vi "Test MultiValue INSERT.vi"(9 "file (use dialog)":path, 10 "Method":T1(ring), 11 "Numeric":i32=1000000) -> (2 "Rows/sec":dbl format="%#_3p", 3 "Time per row":dbl format="%#_3p")   [LabVIEW 2016, in "LV-Data.PGSQL.lvclass"]
uses:
  LV-Data.PGSQL.lvclass
  <vilib>/JDP Science/PostgreSQL Library/Result/PQ Result.lvclass/PQ Result.ctl
  <vilib>/JDP Science/PostgreSQL Library/Connection/Execute Command (No results).vi
  <vilib>/JDP Science/PostgreSQL Library/Result/Clear.vi
  <vilib>/JDP Science/PostgreSQL Library/Connection/Execute Command (Result).vi
  <vilib>/JDP Science/PostgreSQL Library/Connection/Execute (no results).vi
  <vilib>/JDP Science/PostgreSQL Library/Connection/Execute (Return first result with rows).vi
  <vilib>/JDP Science/PostgreSQL Library/Connection/Single Command with parameters.vi
  <userlib>/_OpenG.lib/string/string.llb/Trim Whitespace (String)__ogtk.vi
  <vilib>/JDP Science/PostgreSQL Library/Connection/PQ Connection.lvclass
panel:
  out "concatenated string":string
  in  "Connection Strings to access PostgreSQL":string="host=localhost port=5432 dbname = mydb "
  out "error out":errorcluster
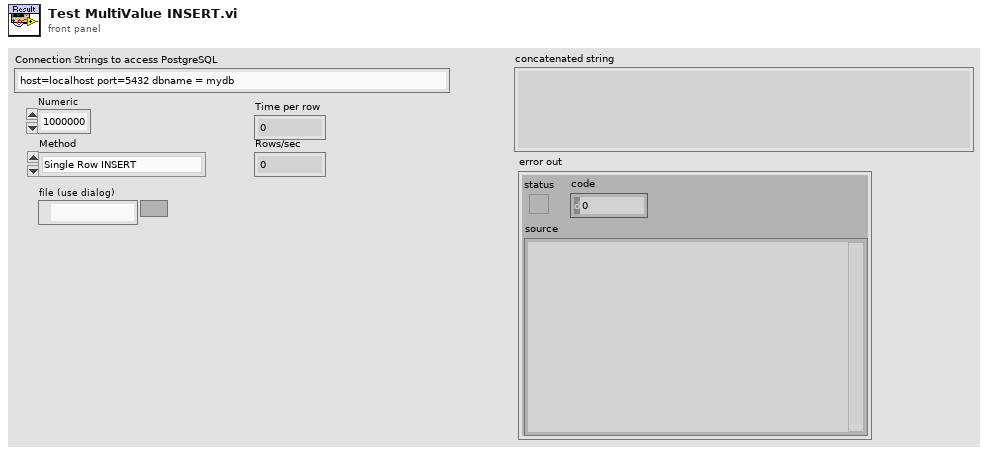
[diagram p1: front panel]
types:
  T1 = enum16{"Single Row INSERT", "Multi Row INSERT", "COPY", "COPY file"}
  T2 = cluster{i32, "number: 0 to 1":dbl, string, "seconds since 1Jan1904":timestamp}
  T3 = typedef "NI_Data Type.lvlib/Data Type.ctl" = enum8{"Invalid Type", "Void", "I8", "I16", "I32", "I64", "U8", "U16", "U32", "U64", "Single Float", "Double Float", "Extended Float", "Single Complex", "Double Complex", "Extended Complex", "Enum U8", "Enum U16", "Enum U32", "Enum U64", "Single Float With Unit", "Double Float With Unit", "Extended Float With Unit", "Single Complex with Unit", "Double Complex with Unit", "Extended Complex with Unit", "Boolean", "String", "Path", "Picture", "Tag", "Array", "Cluster", "Variant", "LV Variant", "Waveform", "Timestamp", "Digital Waveform", "Digital Data", "ExpressData", "Refnum", "External Data", "VI", "Poly VI", "LabVIEW Class Instance", "Fixed Point"}
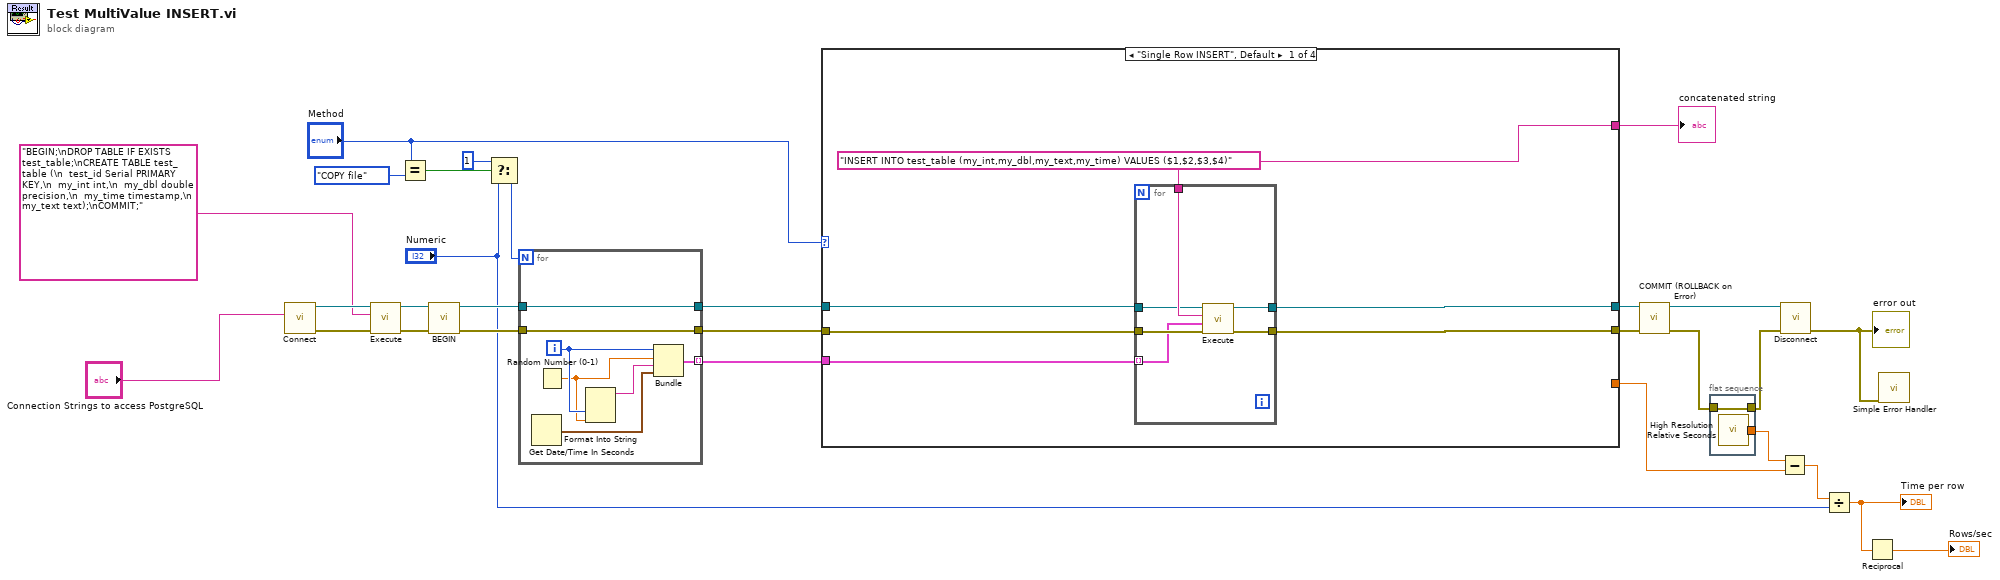
[diagram p0: block diagram]
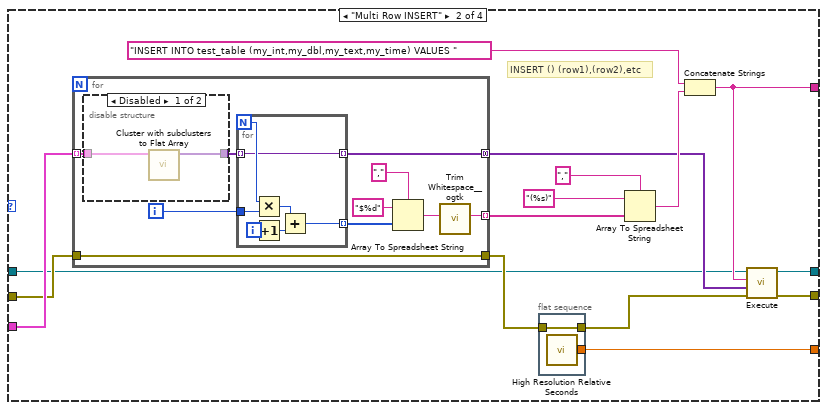
[diagram p2: hidden frame]
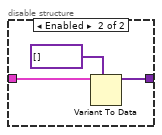
[diagram p3: hidden frame]
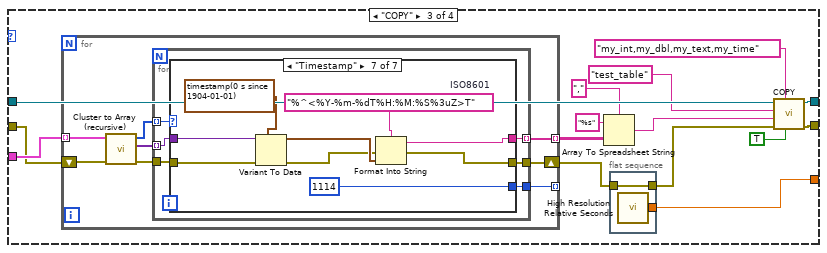
[diagram p4: hidden frame]
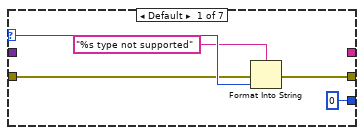
[diagram p5: hidden frame]
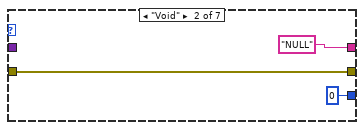
[diagram p6: hidden frame]
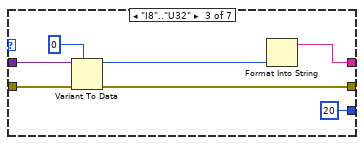
[diagram p7: hidden frame]
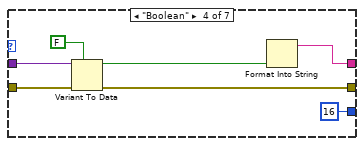
[diagram p8: hidden frame]
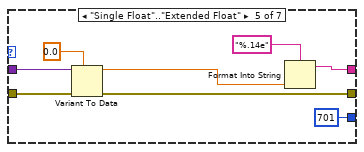
[diagram p9: hidden frame]
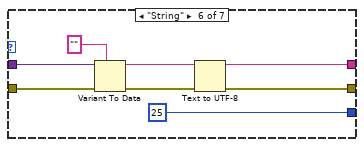
[diagram p10: hidden frame]
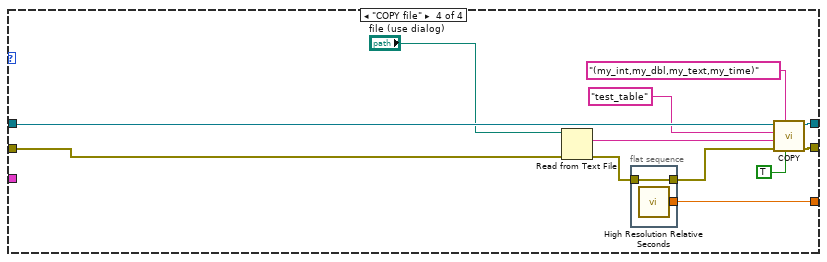
[diagram p11: hidden frame]
diagram:
  n1 = call <vilib>:"Connect.vi"("Connection Strings"="Connection Strings to access PostgreSQL") -> ("error out"=w25:errorcluster, "PQ Connection out"=w27:refnum<class "PQ Connection.lvclass">)  [unwired: 9 in]
  n2 = call-poly <vilib>:"Execute.vi"("error in (no error)"=w25, "SQL"="BEGIN;\nDROP TABLE IF EXISTS test_table;\nCREATE TABLE test_table (\n  test_id Serial PRIMARY KEY,\n  my_int int,\n  my_dbl double precision,\n  my_time timestamp,\n  my_text text);\nCOMMIT;", "PQ Connection in"=w27) -> ("error out"=w10:errorcluster, "PQ Connection out"=w26:refnum<class "PQ Connection.lvclass">)  [unwired: 7 in]
  n3 = Equal?(x="Method", y=T1."COPY file") -> (x = y?=w6:bool)
  n4 = call <vilib>:"BEGIN.vi"("error in (no error)"=w10, "PQ Connection in"=w26) -> ("error out"=w18:errorcluster, "PQ Connection out"=w19:refnum<class "PQ Connection.lvclass">)  [unwired: 8 in]
  n5 = Select(t=1, s=w6, f="Numeric") -> (s? t:f=w5:i32)
  n6 = for {
    N: w5 -> [_]
    tunnel: [w32] -> w11 mode=indexing
    tunnel: w18 -> [w35]
    tunnel: [w35] -> w2
    tunnel: w19 -> [w36]
    tunnel: [w36] -> w15
    i -> [w34]
    n7 = Get Date/Time In Seconds() -> (seconds since 1Jan1904=w31:timestamp)
    n8 = Random Number (0-1)() -> (number: 0 to 1=w33:dbl)
    n9 = Format Into String(w34, w33) -> (resulting string=w30:string)  [unwired: 3 in, 1 out]
    n10 = Bundle(w34, "number: 0 to 1"=w33, w30, "seconds since 1Jan1904"=w31) -> (w32:T2)  [unwired: 1 in]
  }
  n11 = case shown="\"Single Row INSERT\", Default" "Method" {
    tunnel: w11 -> [w38 w63 w98 _]
    tunnel: w15 -> [w41 w49 w102 w177]
    tunnel: [w39 w57 w100 w175] -> w14
    tunnel: [w40 w56 w101 w176] -> w13
    tunnel: w2 -> [w42 w52 w97 w169]
    tunnel: [w37 w55 _ _] -> w12
    tunnel: [_ w50 w88 w166] -> w1
    frame "Single Row INSERT", Default {
      w37 = "INSERT INTO test_table (my_int,my_dbl,my_text,my_time) VALUES ($1,$2,$3,$4)" ("command")
      n12 = for {
        tunnel: w37 -> [w47]
        tunnel: w38 -> [w43] mode=indexing
        tunnel: w41 -> [w46]
        tunnel: [w48] -> w39
        tunnel: w42 -> [w45]
        tunnel: [w44] -> w40
        n13 = call-poly <vilib>:"Execute.vi"("error in (no error)"=w45, "Parameters"=w43, "SQL"=w47, "PQ Connection in"=w46) -> ("error out"=w44:errorcluster, "PQ Connection out"=w48:refnum<class "PQ Connection.lvclass">)  [unwired: 6 in]
      }
    }
    frame "Multi Row INSERT" {
      # "INSERT () (row1),(row2),etc"
      n14 = for {
        tunnel: w63 -> [w75] mode=indexing
        tunnel: [w67] -> w60 mode=indexing
        tunnel: [w68] -> w54 mode=concatenating
        tunnel: w52 -> [w66]
        tunnel: [w66] -> w53
        i -> [w73]
        n15 = disable-structure shown="Disabled" {
          disable-tunnel: w75 -> [w77 w79]
          disable-tunnel: [w76 w78] -> w74
          frame Disabled {
            n16 = call <vilib>:"Cluster with subclusters to Flat Array.vi"("Variant"=w77) -> ("Array of items"=w76:variant[])  [unwired: 8 in, 2 out]
          }
          frame Enabled {
            n17 = Variant To Data(type=variant[] [], Variant=w79) -> (data=w78:variant[])  [unwired: 1 in, 1 out]
          }
        }
        n18 = for {
          N -> [w86]
          tunnel: w74 -> [w82] mode=indexing
          tunnel: w73 -> [w85]
          tunnel: [w83] -> w72 mode=indexing
          tunnel: [w82] -> w68 mode=indexing
          i -> [w87]
          n19 = Multiply(x=w86, y=w85) -> (x*y=w84:i32)
          n20 = Increment(x=w87) -> (x+1=w81:i32)
          n21 = Add(x=w84, y=w81) -> (x+y=w83:i32)
        }
        n22 = Array To Spreadsheet String(delimiter (Tab)=",", array=w72, 3:"$%d" ("format string")) -> (spreadsheet string=w69:string)
        n23 = call-poly <userlib>:"Trim Whitespace__ogtk.vi"("String in"=w69) -> ("String out"=w67:string)  [unwired: 6 in]
      }
      n24 = flat-sequence {
        tunnel: w53 -> [w65]
        tunnel: [w65] -> w51
        tunnel: [w64] -> w50
        frame #0 {
          n25 = call <vilib>:"High Resolution Relative Seconds.vi"() -> ("relative seconds"=w64:dbl)
        }
      }
      n26 = Array To Spreadsheet String(delimiter (Tab)=",", array=w60, 3:"(%s)" ("format string")) -> (spreadsheet string=w58:string)
      n27 = Concatenate Strings("INSERT INTO test_table (my_int,my_dbl,my_text,my_time) VALUES " ("command"), w58) -> (w55:string)
      n28 = call-poly <vilib>:"Execute.vi"("error in (no error)"=w51, "Parameters"=w54, "SQL"=w55, "PQ Connection in"=w49) -> ("error out"=w56:errorcluster, "PQ Connection out"=w57:refnum<class "PQ Connection.lvclass">)  [unwired: 6 in]
    }
    frame "COPY" {
      n29 = for {
        tunnel: [w112] -> w96 mode=indexing
        shift-right: [w111] -> w90
        shift-left: w97 -> [w109]
        tunnel: [w110] -> _ mode=indexing
        tunnel: w98 -> [w108] mode=indexing
        n30 = call <vilib>:"Cluster to Array (recursive).vi"("error in (no error)"=w109, "Variant"=w108) -> ("error out"=w105:errorcluster, "Elements"=w107:variant[], "Types"=w106:T3[])  [unwired: 7 in]
        n31 = for {
          tunnel: [w118] -> w112 mode=indexing
          tunnel: [w117] -> w111
          tunnel: [w116] -> w110
          tunnel: w107 -> [w114] mode=indexing
          tunnel: w106 -> [w115] mode=indexing
          tunnel: w105 -> [w113]
          n32 = case shown="\"Timestamp\"" w115 {
            selector: w115 -> [w123 _ _ _ _ _ _]
            tunnel: w114 -> [_ _ w133 w140 w148 w156 w165]
            tunnel: [_ "NULL" w130 w138 w145 w151 w157] -> w118
            tunnel: w113 -> [w121 w125 w129 w137 w143 w154 w164]
            tunnel: [w120 w125 w128 w136 w142 w149 w158] -> w117
            tunnel: [0 0 20 16 701 25 1114] -> w116
            frame Default {
              n33 = Format Into String(format string="%s type not supported", error in=w121, w123) -> (error out=w120:errorcluster)  [unwired: 1 in, 1 out]
            }
            frame "Void" {
            }
            frame "I8".."U32" {
              n34 = Variant To Data(error in=w129, type=i64 0, Variant=w133) -> (data=w131:i64, error out=w128:errorcluster)
              n35 = Format Into String(w131) -> (resulting string=w130:string)  [unwired: 3 in, 1 out]
            }
            frame "Boolean" {
              n36 = Variant To Data(error in=w137, type=FALSE, Variant=w140) -> (data=w139:bool, error out=w136:errorcluster)
              n37 = Format Into String(w139) -> (resulting string=w138:string)  [unwired: 3 in, 1 out]
            }
            frame "Single Float".."Extended Float" {
              n38 = Variant To Data(error in=w143, type=0.0, Variant=w148) -> (data=w146:dbl, error out=w142:errorcluster)
              n39 = Format Into String(format string="%.14e", w146) -> (resulting string=w145:string)  [unwired: 2 in, 1 out]
            }
            frame "String" {
              n40 = Variant To Data(error in=w154, type="", Variant=w156) -> (data=w152:string, error out=w150:errorcluster)
              n41 = Text to UTF-8(8:w150, 11:w152) -> (0:w149:errorcluster, 3:w151:string)  [unwired: 1 in]
            }
            frame "Timestamp" {
              w161 = "%^<%Y-%m-%dT%H:%M:%S%3uZ>T"  # ISO8601
              n42 = Variant To Data(error in=w164, type=timestamp(0 s since 1904-01-01), Variant=w165) -> (data=w160:timestamp, error out=w159:errorcluster)
              n43 = Format Into String(format string=w161, error in=w159, w160) -> (resulting string=w157:string, error out=w158:errorcluster)  [unwired: 1 in]
            }
          }
        }
      }
      n44 = Array To Spreadsheet String(delimiter (Tab)=",", array=w96, 3:"%s" ("format string")) -> (spreadsheet string=w91:string)
      n45 = flat-sequence {
        tunnel: w90 -> [w104]
        tunnel: [w104] -> w89
        tunnel: [w103] -> w88
        frame #0 {
          n46 = call <vilib>:"High Resolution Relative Seconds.vi"() -> ("relative seconds"=w103:dbl)
        }
      }
      n47 = call <vilib>:"COPY.vi"("CSV?"=TRUE, "column name(s) (empty=ALL)"="my_int,my_dbl,my_text,my_time" ("command"), "error in (no error)"=w89, "buffer"=w91, "table name"="test_table" ("command"), "PQ Connection in"=w102) -> ("error out"=w101:errorcluster, "PQ Connection out"=w100:refnum<class "PQ Connection.lvclass">)  [unwired: 4 in]
    }
    frame "COPY file" {
      n48 = Read from Text File(file (use dialog)="file (use dialog)", error in=w169) -> (text=w171:string, error out=w168:errorcluster)  [unwired: 2 in, 2 out]
      n49 = flat-sequence {
        tunnel: w168 -> [w179]
        tunnel: [w179] -> w167
        tunnel: [w178] -> w166
        frame #0 {
          n50 = call <vilib>:"High Resolution Relative Seconds.vi"() -> ("relative seconds"=w178:dbl)
        }
      }
      n51 = call <vilib>:"COPY.vi"("CSV?"=TRUE, "column name(s) (empty=ALL)"="(my_int,my_dbl,my_text,my_time)" ("command"), "error in (no error)"=w167, "buffer"=w171, "table name"="test_table" ("command"), "PQ Connection in"=w177) -> ("error out"=w176:errorcluster, "PQ Connection out"=w175:refnum<class "PQ Connection.lvclass">)  [unwired: 4 in]
    }
  }
  "concatenated string" <- w12
  n52 = call <vilib>:"COMMIT (ROLLBACK on Error).vi"("error in (no error)"=w13, "PQ Connection in"=w14) -> ("error out"=w22:errorcluster, "PQ Connection out"=w23:refnum<class "PQ Connection.lvclass">)  [unwired: 8 in]
  n53 = flat-sequence {
    tunnel: w22 -> [w181]
    tunnel: [w181] -> w21
    tunnel: [w180] -> w20
    frame #0 {
      n54 = call <vilib>:"High Resolution Relative Seconds.vi"() -> ("relative seconds"=w180:dbl)
    }
  }
  n55 = Subtract(x=w20, y=w1) -> (x-y=w9:dbl)
  n56 = call-dynamic "Disconnect.vi"("error in (no error)"=w21, "PQ Connection in"=w23) -> ("error out"=w28:errorcluster)  [unwired: 9 in]
  "error out" <- w28
  n57 = Divide(x=w9, y="Numeric") -> (x/y=w17:dbl)
  "Time per row" <- w17
  n58 = Reciprocal(x=w17) -> (1/x=→"Rows/sec":dbl)
  n59 = call <vilib>:"Simple Error Handler.vi"("error in (no error)"=w28) -> ()  [unwired: 4 in, 5 out]
